vi "Handle TCP Connection.vi"(4 "Remote Port":u16, 6 "Remote Host":string, 7 "TCPMessageAPI":refnum<class "TCPMessageAPI.lvclass">, 8 "error in (no error)":errorcluster, 9 "Node ID":u32, 10 "Connection State":T1, 11 "Constellation Command Handler in":refnum<class "Constellation Command Handler.lvclass">) -> (0 "error out":errorcluster, 3 "Constellation Command Handler out":refnum<class "Constellation Command Handler.lvclass">)   [LabVIEW 2023, in "VectoScratch.lvlib" / "Constellation Command Handler.lvclass"]
uses:
  Vecto/Connection State.ctl
  Vecto/TCPMessageService/TCPMessageAPI.lvclass
  Constellation Command Handler.lvclass
  Constellation Command Handler.lvclass/Constellation Command Handler.ctl
  Vecto/Vecto.lvlib
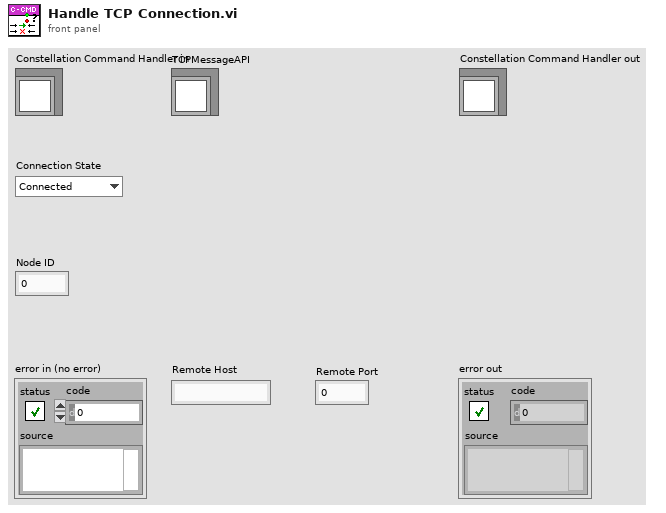
[diagram p1: front panel]
types:
  T1 = typedef "Vecto.lvlib/Connection State.ctl" = enum16{"Connected", "Disconnected"}
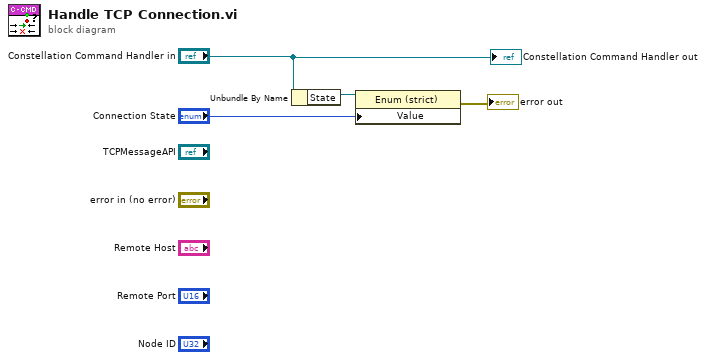
[diagram p0: block diagram]
diagram:
  n1 = Unbundle By Name("Constellation Command Handler in") -> ("State"=w3:refnum<vi>)
  n2 = property class="Enum (strict)"(reference=w3, "Value"="Connection State") -> (error out=→"error out":errorcluster)  [unwired: 1 in, 1 out]
  "Constellation Command Handler out" <- "Constellation Command Handler in"
